vi "2_ExportDatatoExcel.vi"(8 "error in (no error)":errorcluster, 10 "Waveform Graph":waveform(dbl)[](graph), 11 "file path (IN)":path) -> (0 "error out":errorcluster, 3 "file path (OUT)":path)   [LabVIEW 2020]
uses:
  <vilib>/Utility/file.llb/Write Delimited Spreadsheet (string).vi
panel:
  out "Ch4 : Y":dbl[](array[numeric])
  out "Ch4 : appended array":string[](array[string])
  out "Ch3 : Y":dbl[](array[numeric])
  out "Ch3 : appended array":string[](array[string])
  out "Ch2 : Y":dbl[](array[numeric])
  out "Ch2 : appended array":string[](array[string])
  out "Ch1 : appended array":string[](array[string])
  out "Ch1 : Y":dbl[](array[numeric])
  out "dt":dbl
  out "Spread Sheet Display":string[][](array[string])
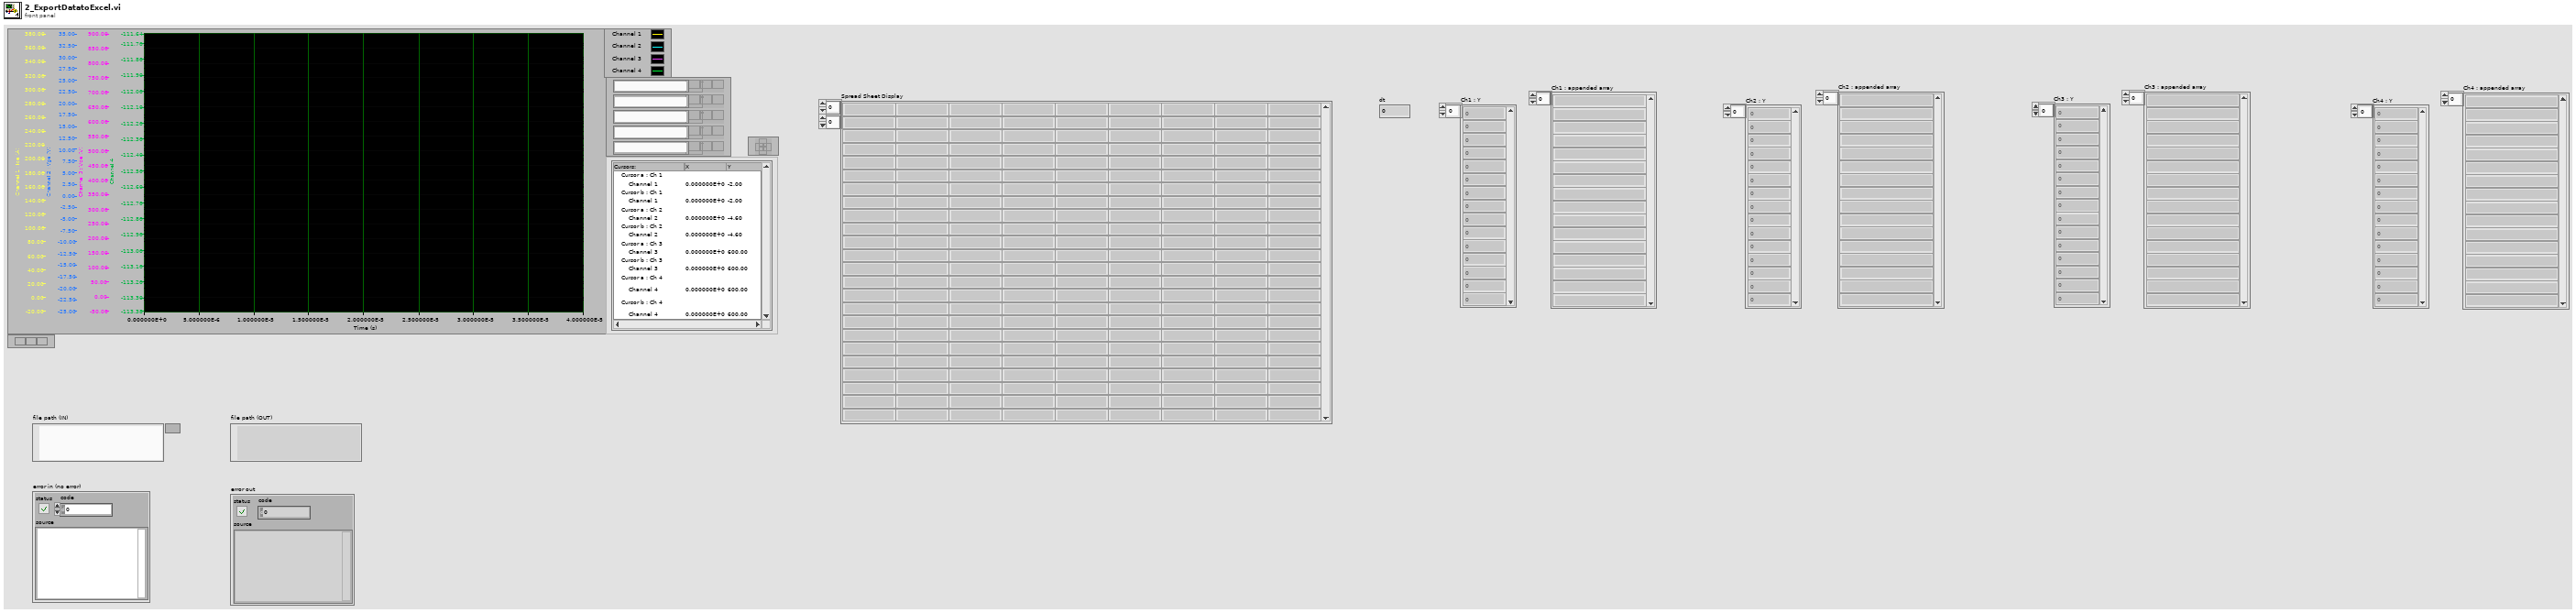
[diagram p1: front panel]
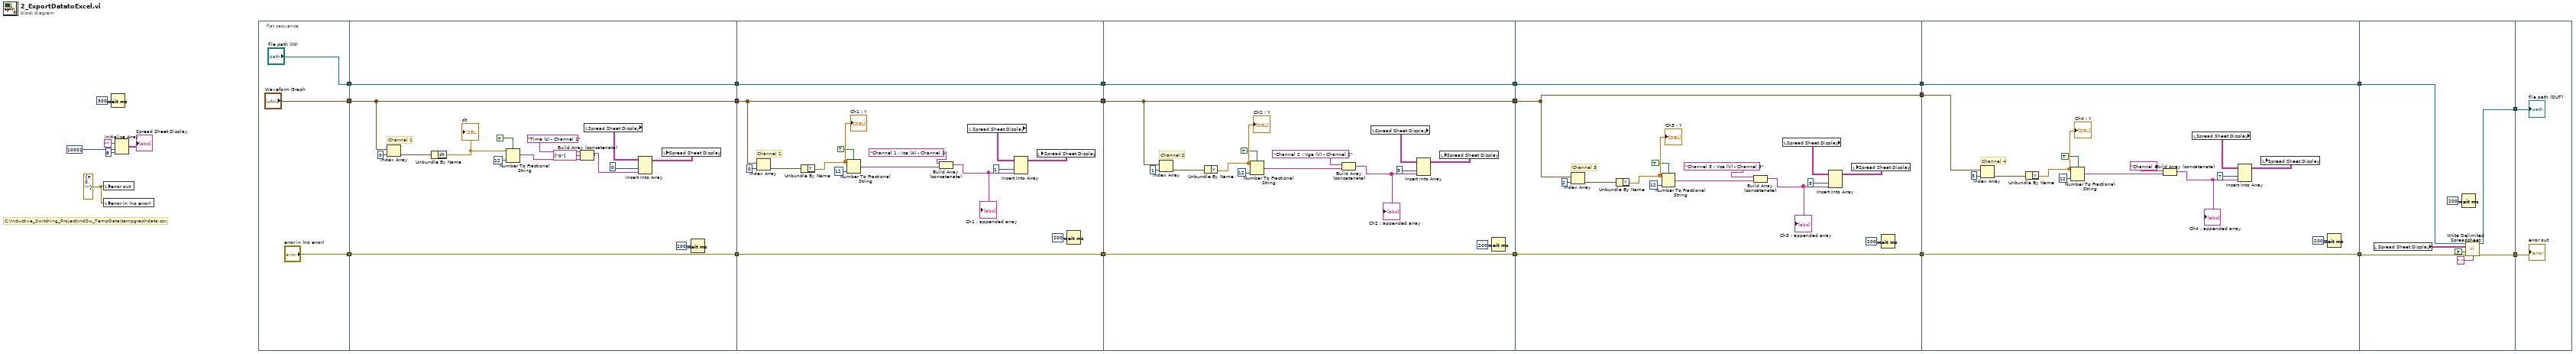
[diagram p0: block diagram]
diagram:
  w11 = errorcluster {"status"=FALSE, "code"=0, "source"=""} ("error out")
  # "C:\\Inductive_Switching_Project\\IndSw_TempData\\tempgraphdata.csv"
  n1 = local write "error out"(w11) -> ()
  n2 = local write "error in (no error)"(w11) -> ()
  n3 = Wait (ms)(milliseconds to wait=u32 300) -> ()  [unwired: 1 out]
  n4 = Initialize Array("", 10001 ("dimension size"), 8 ("dimension size")) -> (→"Spread Sheet Display":string[][])
  n5 = flat-sequence {
    tunnel: ["Waveform Graph"] -> w16
    tunnel: ["error in (no error)"] -> w13
    tunnel: ["file path (IN)"] -> w7
    tunnel: [w32] -> w20
    tunnel: w16 -> [w32]
    tunnel: w13 -> [w31]
    tunnel: [w31] -> w12
    tunnel: [w29] -> w8
    tunnel: w7 -> [w29]
    tunnel: w20 -> [w48]
    tunnel: [w48] -> w19
    tunnel: [w47] -> w14
    tunnel: w12 -> [w47]
    tunnel: [w45] -> w9
    tunnel: w8 -> [w45]
    tunnel: w19 -> [w63]
    tunnel: [w63] -> w18
    tunnel: [w62] -> w15
    tunnel: w14 -> [w62]
    tunnel: [w60] -> w10
    tunnel: w9 -> [w60]
    tunnel: w18 -> [w75]
    tunnel: [w78] -> w5
    tunnel: w15 -> [w78]
    tunnel: [w76] -> w3
    tunnel: w10 -> [w76]
    tunnel: [w75] -> w1
    tunnel: w5 -> [w104]
    tunnel: [w104] -> w4
    tunnel: w3 -> [w103]
    tunnel: [w103] -> w2
    tunnel: w1 -> [w90]
    tunnel: [w109] -> w17
    tunnel: w4 -> [w108]
    tunnel: w2 -> [w106]
    tunnel: [w105] -> w6
    tunnel: w17 -> [w114]
    tunnel: w6 -> [w113]
    frame #0 {
    }
    frame #1 {
      # "Channel 1"
      n6 = Index Array(array=w32, index=0) -> (element=w43:waveform(dbl))
      n7 = Unbundle By Name(w43) -> ("dt"=w41:dbl)
      "dt" <- w41
      n8 = Number To Fractional String(use system decimal point (T)=TRUE, number=w41, precision (6)=i16 12) -> (F-format string=w36:string)  [unwired: 1 in]
      n9 = Build Array (concatenate)("Time (s) - Channel 1", string[] ["0"] ("array"), w36) -> (w35:string[])
      n10 = local read "Spread Sheet Display"() -> (w40:string[][])
      n11 = Insert Into Array(array=w40, index (col)=0 ("disabled index (col)"), new element=w35) -> (w44:string[][])  [unwired: 1 in]
      n12 = local write "Spread Sheet Display"(w44) -> ()
      n13 = Wait (ms)(milliseconds to wait=u32 200) -> ()  [unwired: 1 out]
    }
    frame #2 {
      # "Channel 1"
      n14 = Index Array(array=w48, index=0) -> (element=w55:waveform(dbl))
      n15 = Unbundle By Name(w55) -> ("Y"=w56:dbl[])
      "Ch1 : Y" <- w56
      n16 = Number To Fractional String(use system decimal point (T)=TRUE, number=w56, precision (6)=i16 12) -> (F-format string=w58:string[])  [unwired: 1 in]
      n17 = Build Array (concatenate)("Channel 1 : Ice (A) - Channel 1", w58) -> (w59:string[])
      "Ch1 : appended array" <- w59
      n18 = local read "Spread Sheet Display"() -> (w57:string[][])
      n19 = Insert Into Array(array=w57, index (col)=1 ("disabled index (col)"), new element=w59) -> (w54:string[][])  [unwired: 1 in]
      n20 = local write "Spread Sheet Display"(w54) -> ()
      n21 = Wait (ms)(milliseconds to wait=u32 200) -> ()  [unwired: 1 out]
    }
    frame #3 {
      # "Channel 2"
      n22 = Index Array(array=w63, index=1) -> (element=w74:waveform(dbl))
      n23 = Unbundle By Name(w74) -> ("Y"=w73:dbl[])
      "Ch2 : Y" <- w73
      n24 = Number To Fractional String(use system decimal point (T)=TRUE, number=w73, precision (6)=i16 12) -> (F-format string=w71:string[])  [unwired: 1 in]
      n25 = Build Array (concatenate)("Channel 2 : Vge (V) - Channel 2", w71) -> (w70:string[])
      "Ch2 : appended array" <- w70
      n26 = local read "Spread Sheet Display"() -> (w72:string[][])
      n27 = Insert Into Array(array=w72, index (col)=3 ("disabled index (col)"), new element=w70) -> (w69:string[][])  [unwired: 1 in]
      n28 = local write "Spread Sheet Display"(w69) -> ()
      n29 = Wait (ms)(milliseconds to wait=u32 200) -> ()  [unwired: 1 out]
    }
    frame #4 {
      # "Channel 3"
      n30 = Index Array(array=w75, index=2) -> (element=w85:waveform(dbl))
      n31 = Unbundle By Name(w85) -> ("Y"=w86:dbl[])
      "Ch3 : Y" <- w86
      n32 = Number To Fractional String(use system decimal point (T)=TRUE, number=w86, precision (6)=i16 12) -> (F-format string=w88:string[])  [unwired: 1 in]
      n33 = Build Array (concatenate)("Channel 3 : Vce (V) - Channel 3", w88) -> (w89:string[])
      "Ch3 : appended array" <- w89
      n34 = local read "Spread Sheet Display"() -> (w87:string[][])
      n35 = Insert Into Array(array=w87, index (col)=5 ("disabled index (col)"), new element=w89) -> (w84:string[][])  [unwired: 1 in]
      n36 = local write "Spread Sheet Display"(w84) -> ()
      n37 = Wait (ms)(milliseconds to wait=u32 200) -> ()  [unwired: 1 out]
    }
    frame #5 {
      # "Channel 4"
      n38 = Index Array(array=w90, index=3) -> (element=w96:waveform(dbl))
      n39 = Unbundle By Name(w96) -> ("Y"=w95:dbl[])
      "Ch4 : Y" <- w95
      n40 = Number To Fractional String(use system decimal point (T)=TRUE, number=w95, precision (6)=i16 12) -> (F-format string=w93:string[])  [unwired: 1 in]
      n41 = Build Array (concatenate)("Channel 4", w93) -> (w92:string[])
      "Ch4 : appended array" <- w92
      n42 = local read "Spread Sheet Display"() -> (w94:string[][])
      n43 = Insert Into Array(array=w94, index (col)=7 ("disabled index (col)"), new element=w92) -> (w97:string[][])  [unwired: 1 in]
      n44 = local write "Spread Sheet Display"(w97) -> ()
      n45 = Wait (ms)(milliseconds to wait=u32 200) -> ()  [unwired: 1 out]
    }
    frame #6 {
      n46 = local read "Spread Sheet Display"() -> (w112:string[][])
      n47 = Wait (ms)(milliseconds to wait=u32 200) -> ()  [unwired: 1 out]
      n48 = call-poly <vilib>:"Write Delimited Spreadsheet.vi"("file path (dialog if empty)"=w106, "2D data"=w112, "append to file? (new file:F)"=FALSE, "error in (no error)"=w108, "delimiter (\\t)"="," ("delimiter (\\t)")) -> ("new file path (Not A Path if cancelled)"=w105:path, "error out"=w109:errorcluster)  [unwired: 9 in]
    }
    frame #7 {
      "error out" <- w114
      "file path (OUT)" <- w113
    }
  }
